vi "InitialiseProbeplan.vi"() -> ()   [LabVIEW 2013]
doc: "General utility to initialise, generate, test and execute probe plans."
uses:
  ProbePlanParams.vi
  InstrControl/ProbeStationControl/ProbeStationControl.lvclass
  general_VIs/globals/QC_MeasurementSetup.vi
panel:
  in  "Continue":bool
  in  "New Sensor":bool
  in  "Single Needle":bool
  out "Chuck Up/Down check":bool
  in  "Probe Card Channels":i32=32
  in  "Strip No.":u16(ring)
  out "Probeplan:":string
  in  "Region":u16(ring)
  in  "Chuck":bool caption="Chuck\nDOWN"
  in  "New Button":bool
  in  "Jump Button":bool
  # "Probeplan"
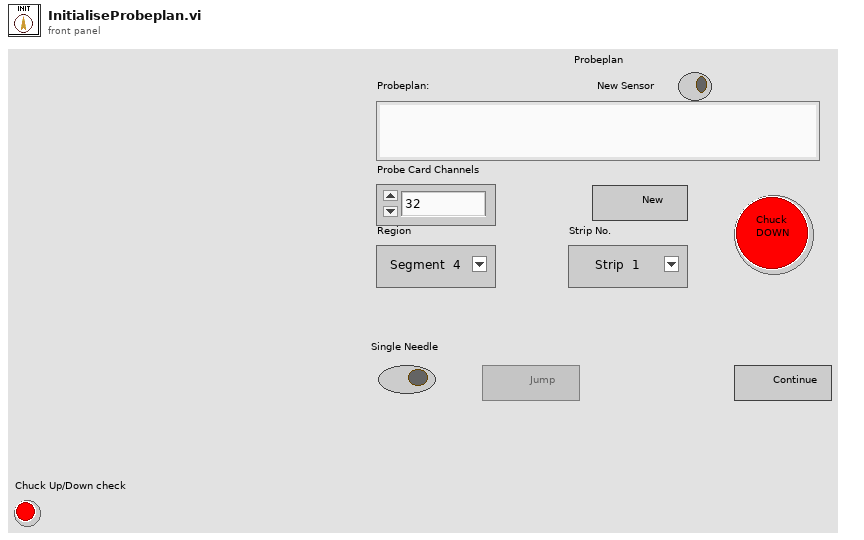
[diagram p1: front panel]
types:
  T1 = cluster{"Bias Supply":refnum<class "SupplyControl.lvclass">, "SMU":refnum<class "SupplyControl.lvclass">, "LCR":refnum<class "LCRControl.lvclass">, "Probe Card Channels":i32, "Bias Voltage [V]":dbl, "First strip":i32, "Last strip":i32, "Base Voltage [V]":dbl, "Base Ramp Step [V]":dbl, "Base Ramp Interval [ms]":u32, "High Voltage [V]":dbl, "High Ramp Step [V]":dbl, "High Ramp Interval [ms]":u32, "Single Needle":bool, "Temperature Readout":enum16{"Read Arduino", "Enter manually"}, "Arduino":refnum<class "ArduinoControl.lvclass">, "Fraction of good strips [%]":dbl, "ProbeStation":refnum<class "ProbeStationControl.lvclass">, "AC frequency [Hz]":i32, "Switching":refnum<class "Switching.lvclass">, "Matrix used?":bool, "Matrix X Channels":cluster{"Bias Supply / SMU LO":i32, "Bias Supply / SMU HI":i32, "CV Box LO":i32, "CV Box HI":i32, "CV Box LO IN":i32, "CV Box HI IN":i32, "Volt meter LO":i32, "Volt meter HI":i32, "Mux1 C1":i32, "Mux1 C2":i32, "Mux2 C1":i32, "Mux2 C2":i32}, "Pinholes Y/N":bool, "Capacitance Y/N":bool, "Resistance Y/N":bool}
  T2 = cluster{"Strip Number OUT":i32, "X0":i32, "Y0":i32, "X1":i32, "Y1":i32, "Xref":dbl, "Yref":dbl, "ProbePlan type":u32, "Inner pads offset":ext, "Outer pads offset":ext, "l_inner":ext, "l_outer":ext, "strip numbering":u16, "Device Orientation":ext, "Stagger offset":i32, "Yoffset":dbl, "Strip pitch":dbl, "Fiducail separation":dbl, "Radius":ext, "Relative strip angles":dbl, "Probeplan description":string, "ProbePlan array":cluster{"Region":string, "ProbePoints":cluster{"X":dbl, "Y":dbl, "Label":string, "CardViable?":bool}[]}[], "Test ProbePoints":cluster{"Regions Enabled":bool[], "From index":u32[], "To index":u32[]}}
  T3 = cluster{"Region":string, "ProbePoints":cluster{"X":dbl, "Y":dbl, "Label":string, "CardViable?":bool}[]}[]
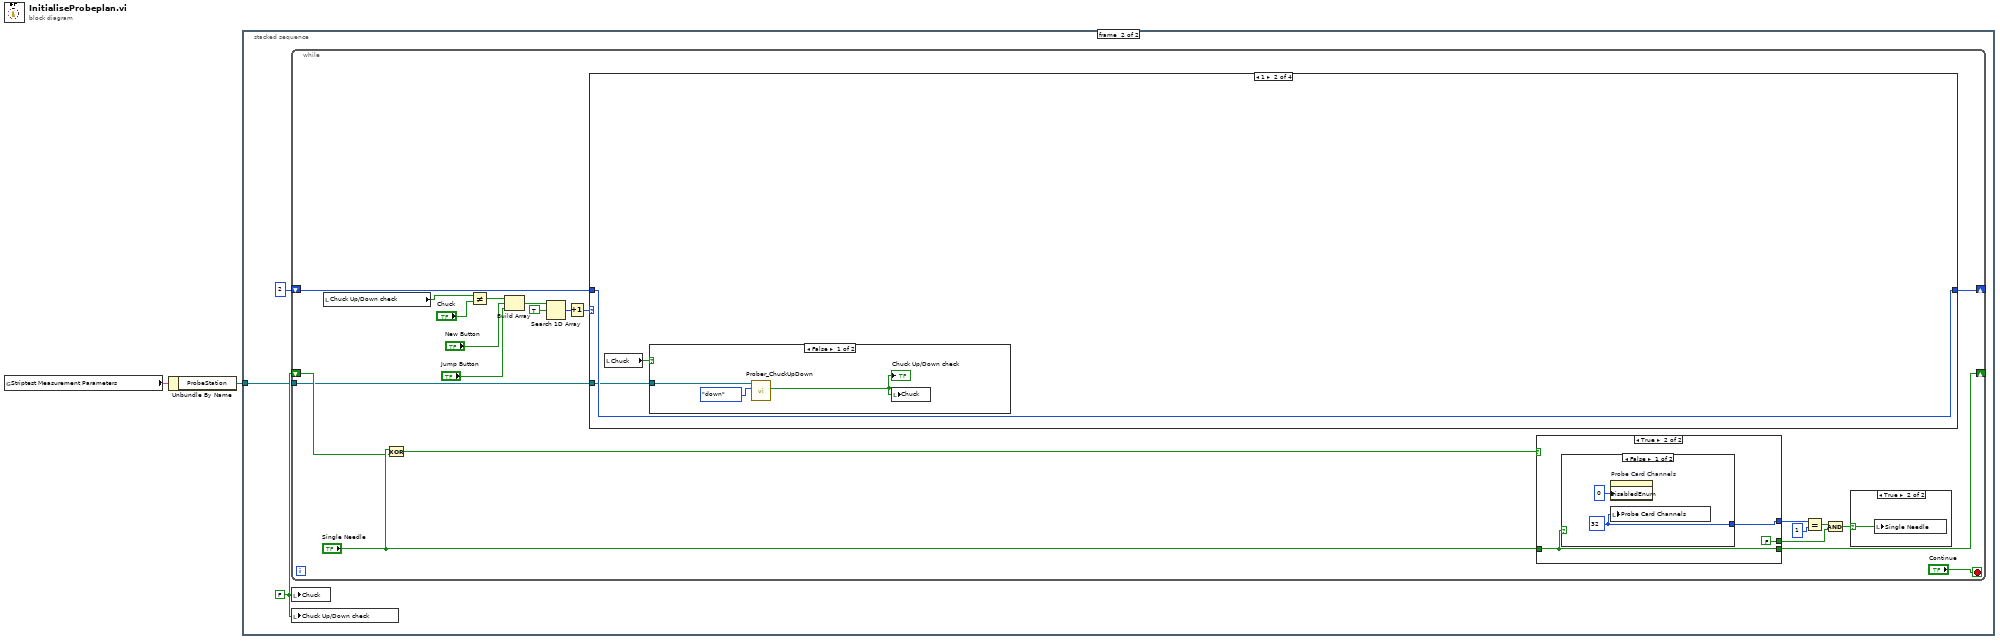
[diagram p0: block diagram]
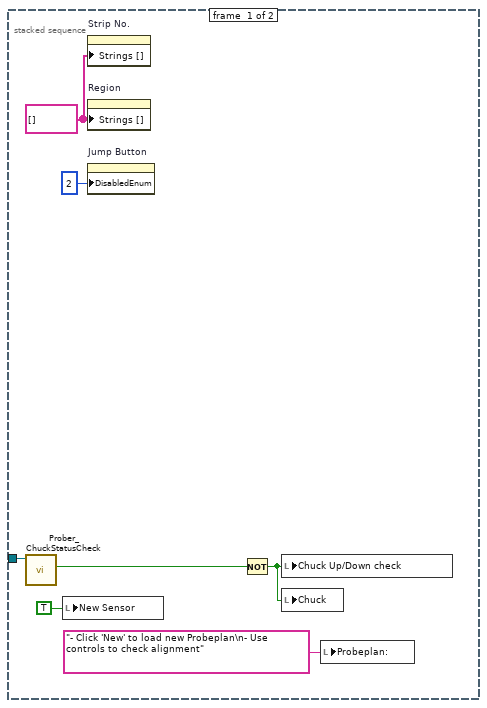
[diagram p2: hidden frame]
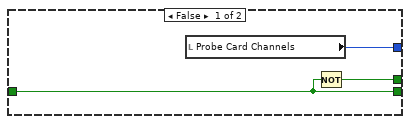
[diagram p4: hidden frame]
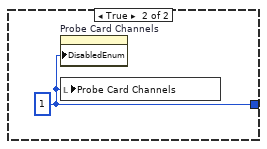
[diagram p5: hidden frame]
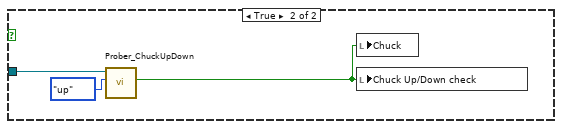
[diagram p7: hidden frame]
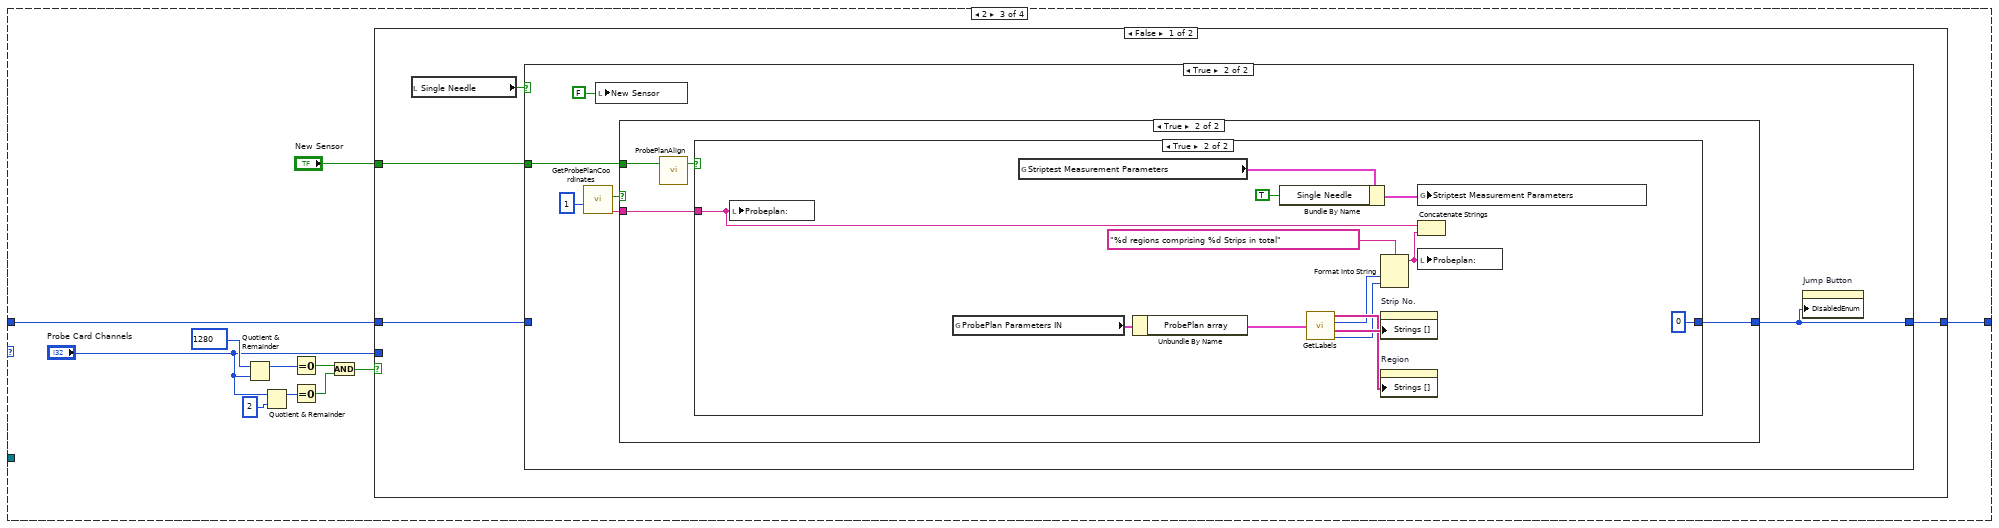
[diagram p8: hidden frame]
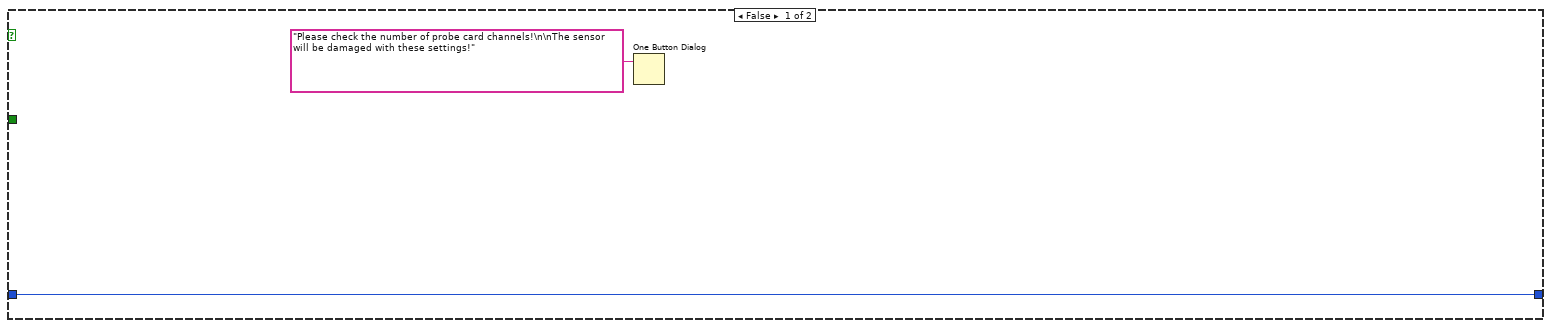
[diagram p9: hidden frame]
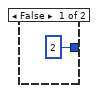
[diagram p10: hidden frame]
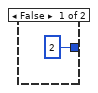
[diagram p11: hidden frame]
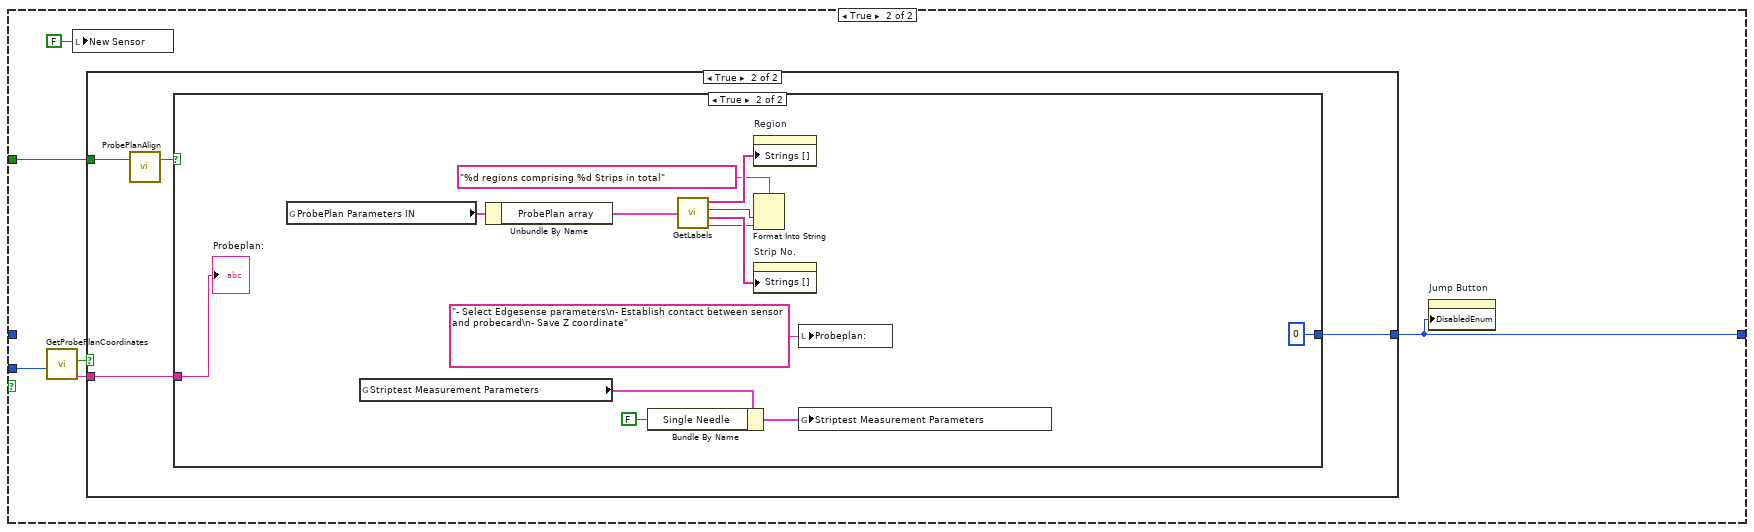
[diagram p12: hidden frame]
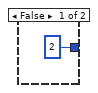
[diagram p13: hidden frame]
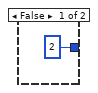
[diagram p14: hidden frame]
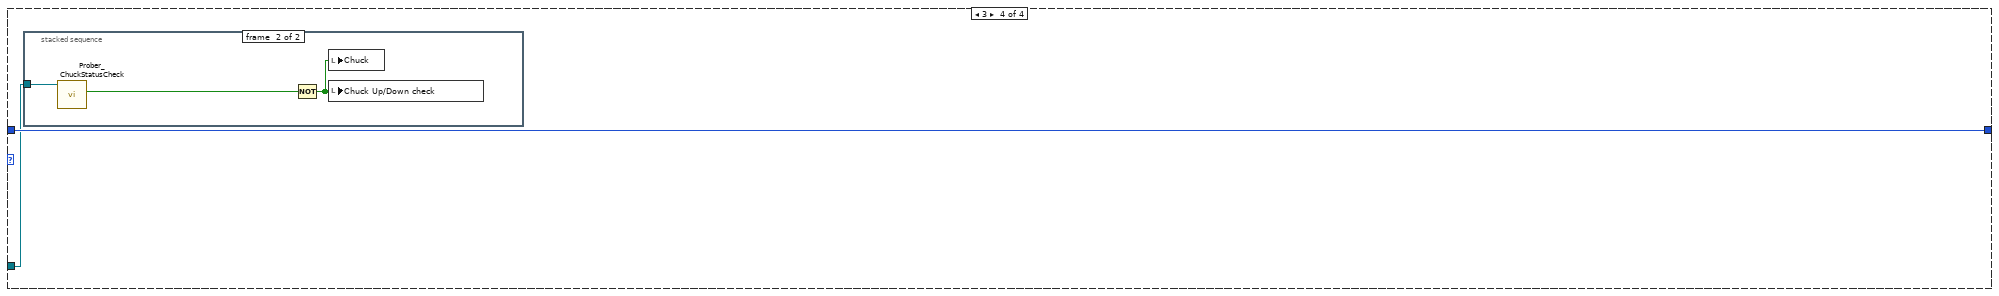
[diagram p15: hidden frame]
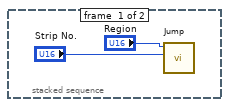
[diagram p16: hidden frame]
diagram:
  n1 = global read "QC_MeasurementSetup.vi" "Striptest Measurement Parameters"() -> (w2:T1)
  n2 = Unbundle By Name(w2) -> ("ProbeStation"=w1:refnum<class "ProbeStationControl.lvclass">)
  n3 = stacked-sequence {
    tunnel: w1 -> [w3 w10]
    frame #0 {
      w7 = string[] []
      n4 = call-dynamic "Prober_ChuckStatusCheck.vi"("ProbeStationControl in"=w3) -> ("Chuck at CONTACT?"=w5:bool)  [unwired: 8 in, 2 out]
      n5 = local write "New Sensor"(TRUE) -> ()
      n6 = property on="Strip No." class="Ring (strict)"("Strings []"=w7) -> ()  [unwired: 2 in, 2 out]
      n7 = property on="Region" class="Ring (strict)"("Strings []"=w7) -> ()  [unwired: 2 in, 2 out]
      n8 = property on="Jump Button" class="Bool"("DisabledEnum"=2) -> ()  [unwired: 2 in, 2 out]
      n9 = Not(x=w5) -> (.not. x?=w4:bool)
      n10 = local write "Chuck Up/Down check"(w4) -> ()
      n11 = local write "Chuck"(w4) -> ()
      n12 = local write "Probeplan:"("- Click 'New' to load new Probeplan\n- Use controls to check alignment") -> ()
    }
    frame #1 {
      w11 = FALSE
      n13 = while {
        shift-right: [w27] -> _
        shift-left: 2 -> [w28]
        shift-right: [w15] -> _
        shift-left: w11 -> [w16]
        tunnel: w10 -> [w13]
        stop <- "Continue" stop-if-true
        n14 = local read "Chuck Up/Down check"() -> (w26:bool)
        n15 = Exclusive Or(1:w16, 2:"Single Needle") -> (0:w18:bool)
        n16 = Not Equal?(x=w26, y="Chuck") -> (x != y?=w24:bool)
        n17 = Build Array(w24, "New Button", "Jump Button") -> (w33:bool[])
        n18 = Search 1D Array(1D array=w33, element=TRUE) -> (index of element=w34:i32)  [unwired: 1 in]
        n19 = Increment(x=w34) -> (x+1=w29:i32)
        n20 = case shown="1" w29 {
          tunnel: w28 -> [w45 w48 w63 w123]
          tunnel: [w45 w48 w65 w123] -> w27
          tunnel: w13 -> [_ w46 _ w122]
          frame 0, Default {
          }
          frame 1 {
            n21 = local read "Chuck"() -> (w47:bool)
            n22 = case shown="False" w47 {
              tunnel: w46 -> [w50 w52]
              frame False {
                n23 = call-dynamic "Prober_ChuckUpDown.vi"("Direction"=enum16{"up", "down"}."down", "ProbeStationControl in"=w50) -> ("Chuck at CONTACT?"=w51:bool)  [unwired: 7 in, 2 out]
                "Chuck Up/Down check" <- w51
                n24 = local write "Chuck"(w51) -> ()
              }
              frame True {
                n25 = call-dynamic "Prober_ChuckUpDown.vi"("Direction"=enum16{"up", "down"}."up", "ProbeStationControl in"=w52) -> ("Chuck at CONTACT?"=w54:bool)  [unwired: 7 in, 2 out]
                n26 = local write "Chuck"(w54) -> ()
                n27 = local write "Chuck Up/Down check"(w54) -> ()
              }
            }
          }
          frame 2 {
            n28 = Quotient & Remainder(x=1280, y="Probe Card Channels") -> (x-y*floor(x/y)=w64:i32)  [unwired: 1 out]
            n29 = Quotient & Remainder(x="Probe Card Channels", y=2) -> (x-y*floor(x/y)=w57:i32)  [unwired: 1 out]
            n30 = Equal To 0?(x=w64) -> (x = 0?=w62:bool)
            n31 = Equal To 0?(x=w57) -> (x = 0?=w56:bool)
            n32 = And(x=w62, y=w56) -> (x .and. y?=w61:bool)
            n33 = case shown="False" w61 {
              tunnel: "Probe Card Channels" -> [_ w100]
              tunnel: [w68 w99] -> w65
              tunnel: w63 -> [w67 _]
              tunnel: "New Sensor" -> [w66 w98]
              frame False {
                n34 = local read "Single Needle"() -> (w69:bool)
                n35 = case shown="True" w69 {
                  tunnel: [w70 w74] -> w68
                  tunnel: w67 -> [w70 _]
                  tunnel: w66 -> [_ w73]
                  frame False {
                    n36 = One Button Dialog(message="Please check the number of probe card channels!\n\nThe sensor will be damaged with these settings!") -> ()  [unwired: 1 in, 1 out]
                  }
                  frame True {
                    n37 = call "GetProbePlanCoordinates.vi"("Probe Card Channels"=1) -> ("file path"=w76:string, "OK?"=w77:bool)  [unwired: 1 out]
                    n38 = local write "New Sensor"(FALSE) -> ()
                    n39 = case shown="True" w77 {
                      tunnel: [2 w82] -> w74
                      tunnel: w76 -> [_ w80]
                      tunnel: w73 -> [_ w79]
                      frame False {
                      }
                      frame True {
                        n40 = call "ProbePlanAlign.vi"("New Sensor"=w79) -> ("Accept/Quit"=w81:bool)  [unwired: 2 in]
                        n41 = case shown="True" w81 {
                          tunnel: [2 0] -> w82
                          tunnel: w80 -> [_ w85]
                          frame False {
                          }
                          frame True {
                            n42 = local write "Probeplan:"(w85) -> ()
                            n43 = global read "ProbePlanParams.vi" "ProbePlan Parameters IN"() -> (w95:T2)
                            n44 = global read "QC_MeasurementSetup.vi" "Striptest Measurement Parameters"() -> (w87:T1)
                            n45 = Unbundle By Name(w95) -> ("ProbePlan array"=w94:T3)
                            n46 = Bundle By Name(cluster=w87, "Single Needle"=TRUE) -> (w86:T1)
                            n47 = call "GetLabels.vi"("Array"=w94) -> ("Region Labels"=w92:string[], "No. of regions"=w91:i32, "Strip Labels"=w93:string[], "No. of Points"=w90:i32)
                            n48 = Format Into String(format string="%d regions comprising %d Strips in total", w91, w90) -> (resulting string=w84:string)  [unwired: 2 in, 1 out]
                            n49 = property on="Strip No." class="Ring (strict)"("Strings []"=w93) -> ()  [unwired: 2 in, 2 out]
                            n50 = property on="Region" class="Ring (strict)"("Strings []"=w92) -> ()  [unwired: 2 in, 2 out]
                            n51 = global write "QC_MeasurementSetup.vi" "Striptest Measurement Parameters"(w86) -> ()
                            n52 = Concatenate Strings(w85, w84) -> ()  [unwired: 1 out]
                            n53 = local write "Probeplan:"(w84) -> ()
                          }
                        }
                      }
                    }
                    n54 = property on="Jump Button" class="Bool"("DisabledEnum"=w74) -> ()  [unwired: 2 in, 2 out]
                  }
                }
              }
              frame True {
                n55 = call "GetProbePlanCoordinates.vi"("Probe Card Channels"=w100) -> ("file path"=w101:string, "OK?"=w102:bool)  [unwired: 1 out]
                n56 = local write "New Sensor"(FALSE) -> ()
                n57 = case shown="True" w102 {
                  tunnel: [2 w107] -> w99
                  tunnel: w101 -> [_ w105]
                  tunnel: w98 -> [_ w104]
                  frame False {
                  }
                  frame True {
                    n58 = call "ProbePlanAlign.vi"("New Sensor"=w104) -> ("Accept/Quit"=w106:bool)  [unwired: 2 in]
                    n59 = case shown="True" w106 {
                      tunnel: [2 0] -> w107
                      tunnel: w105 -> [_ w120]
                      frame False {
                      }
                      frame True {
                        n60 = global read "ProbePlanParams.vi" "ProbePlan Parameters IN"() -> (w119:T2)
                        n61 = global read "QC_MeasurementSetup.vi" "Striptest Measurement Parameters"() -> (w110:T1)
                        n62 = Unbundle By Name(w119) -> ("ProbePlan array"=w118:T3)
                        n63 = Bundle By Name(cluster=w110, "Single Needle"=FALSE) -> (w109:T1)
                        n64 = call "GetLabels.vi"("Array"=w118) -> ("Region Labels"=w116:string[], "No. of regions"=w115:i32, "Strip Labels"=w117:string[], "No. of Points"=w114:i32)
                        n65 = property on="Region" class="Ring (strict)"("Strings []"=w116) -> ()  [unwired: 2 in, 2 out]
                        n66 = Format Into String(format string="%d regions comprising %d Strips in total", w115, w114) -> ()  [unwired: 2 in, 2 out]
                        n67 = property on="Strip No." class="Ring (strict)"("Strings []"=w117) -> ()  [unwired: 2 in, 2 out]
                        n68 = local write "Probeplan:"("- Select Edgesense parameters\n- Establish contact between sensor and probecard\n- Save Z coordinate") -> ()
                        n69 = global write "QC_MeasurementSetup.vi" "Striptest Measurement Parameters"(w109) -> ()
                        "Probeplan:" <- w120
                      }
                    }
                  }
                }
                n70 = property on="Jump Button" class="Bool"("DisabledEnum"=w99) -> ()  [unwired: 2 in, 2 out]
              }
            }
          }
          frame 3 {
            n71 = stacked-sequence {
              tunnel: w122 -> [_ w126]
              frame #0 {
                n72 = call "Jump.vi"("Strip No."="Strip No.", "Region"="Region") -> ()  [unwired: 5 in, 1 out]
              }
              frame #1 {
                n73 = call-dynamic "Prober_ChuckStatusCheck.vi"("ProbeStationControl in"=w126) -> ("Chuck at CONTACT?"=w128:bool)  [unwired: 8 in, 2 out]
                n74 = Not(x=w128) -> (.not. x?=w127:bool)
                n75 = local write "Chuck"(w127) -> ()
                n76 = local write "Chuck Up/Down check"(w127) -> ()
              }
            }
          }
        }
        n77 = case shown="True" w18 {
          tunnel: [w37 FALSE] -> w21
          tunnel: [w38 w40] -> w19
          tunnel: "Single Needle" -> [w36 w39]
          tunnel: [w36 w39] -> w15
          frame False {
            n78 = local read "Probe Card Channels"() -> (w38:i32)
            n79 = Not(x=w36) -> (.not. x?=w37:bool)
          }
          frame True {
            n80 = case shown="False" w39 {
              tunnel: [w42 w44] -> w40
              frame False {
                w42 = 32
                n81 = property on="Probe Card Channels" class="DigNum (strict)"("DisabledEnum"=0) -> ()  [unwired: 2 in, 2 out]
                n82 = local write "Probe Card Channels"(w42) -> ()
              }
              frame True {
                w44 = 1
                n83 = property on="Probe Card Channels" class="DigNum (strict)"("DisabledEnum"=w44) -> ()  [unwired: 2 in, 2 out]
                n84 = local write "Probe Card Channels"(w44) -> ()
              }
            }
          }
        }
        n85 = Equal?(x=w19, y=1) -> (x = y?=w22:bool)
        n86 = And(x=w22, y=w21) -> (x .and. y?=w20:bool)
        n87 = case shown="True" w20 {
          selector: w20 -> [_ w35]
          frame False {
          }
          frame True {
            n88 = local write "Single Needle"(w35) -> ()
          }
        }
      }
      n89 = local write "Chuck"(w11) -> ()
      n90 = local write "Chuck Up/Down check"(w11) -> ()
    }
  }
